vi "Flash Start Live Mode.vi"(8 "error in (no error)":errorcluster, 10 "Camera Settings":T1={"Exposure Time (ms)"=100.0, "Binning"=enum."2x2", "Scan Mode (Flash)"=enum."Fast", "Trigger Mode (Flash)"=enum."Fast", "Frames to Acquire"=1000.0, "Pixel Correction (Flash)"=FALSE} {"Exposure Time (ms)" min=1.0 max=10000.0 step=1.0}, 11 "Orca-Flash 4.0 V2 in":refnum<class "Orca-Flash 4.0 V2.lvclass">) -> (0 "error out":errorcluster, 3 "Orca-Flash 4.0 V2 out":refnum<class "Orca-Flash 4.0 V2.lvclass">)   [LabVIEW 2018, in "Orca-Flash 4.0 V2.lvlib" / "Orca-Flash 4.0 V2.lvclass"]
uses:
  Orca-Flash 4.0 V2.lvclass
  C:/LVCUR/flash-gordon/Hardware/Camera/Camera.lvclass
  Resources/Type Defs/Camera Settings.ctl
  Orca-Flash 4.0 V2.lvclass/Orca-Flash 4.0 V2.ctl
  Resources/GLOBAL/GLOBAL Time-critical.vi
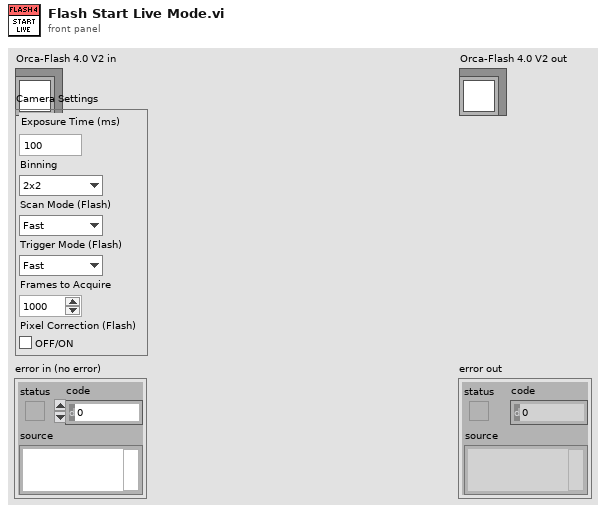
[diagram p1: front panel]
types:
  T1 = typedef "Camera Settings.ctl" = cluster{"Exposure Time (ms)":dbl, "Binning":enum16{"1x1", "2x2", "4x4"}, "Scan Mode (Flash)":enum16{"Fast", "Slow"}, "Trigger Mode (Flash)":enum16{"Fast", "Standard"}, "Frames to Acquire":dbl, "Pixel Correction (Flash)":bool}
  T2 = cluster{"height":i32, "width":i32, "datatype":i32}
  T3 = typedef "Semaphore RefNum" = refnum<k1>
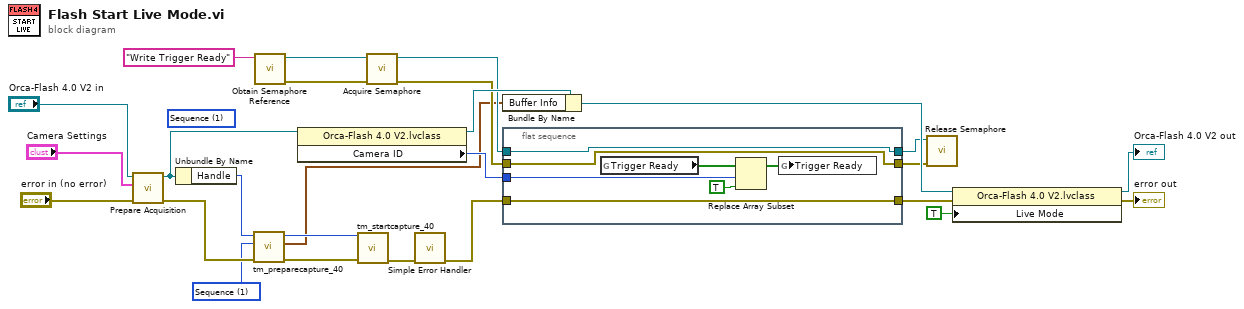
[diagram p0: block diagram]
diagram:
  w4 = 1 items=["Snap", "Sequence"] ("Capture mode")
  (unwired) 1 items=["Snap", "Sequence"] ("Capture mode")
  n1 = call "Prepare Acquisition.vi"("error in (no error)"="error in (no error)", "Flash Settings"="Camera Settings", "Orca-Flash 4.0 in"="Orca-Flash 4.0 V2 in") -> ("error out"=w6:errorcluster, "Orca-Flash 4.0 out"=w16:refnum<class "Orca-Flash 4.0 V2.lvclass">)  [unwired: 7 in]
  n2 = Unbundle By Name(w16) -> ("Handle"=w5:u32)
  n3 = call <userlib>:"tm_preparecapture_40.vi"("error in (no error)"=w6, "Capture mode"=w4, "Handle in"=w5) -> ("error out"=w8:errorcluster, "Buffer Info"=w3:T2, "Handle out"=w7:u32)  [unwired: 5 in, 1 out]
  n4 = call <vilib>:"Obtain Semaphore Reference.vi"("name (unnamed)"="Write Trigger Ready") -> ("error out"=w13:errorcluster, "semaphore"=w14:T3)  [unwired: 4 in, 1 out]
  n5 = property class="Orca-Flash 4.0 V2.lvclass"(reference=w16) -> (reference out=w17:refnum<class "Orca-Flash 4.0 V2.lvclass">, "Camera ID"=w19:i32)  [unwired: 1 in, 1 out]
  n6 = call <userlib>:"tm_startcapture_40.vi"("error in (no error)"=w8, "Handle in"=w7) -> ("error out"=w2:errorcluster)  [unwired: 8 in, 1 out]
  n7 = call <vilib>:"Acquire Semaphore.vi"("error in (no error)"=w13, "semaphore"=w14) -> ("error out"=w9:errorcluster, "semaphore out"=w10:T3)  [unwired: 3 in, 1 out]
  n8 = call <vilib>:"Simple Error Handler.vi"("error in (no error)"=w2) -> ("error out"=w1:errorcluster)  [unwired: 4 in, 4 out]
  n9 = Bundle By Name(cluster=w17, "Buffer Info"=w3) -> (w23:refnum<class "Orca-Flash 4.0 V2.lvclass">)
  n10 = flat-sequence {
    tunnel: w1 -> [w33]
    tunnel: [w33] -> w20
    tunnel: w19 -> [w30]
    tunnel: [w28] -> w12
    tunnel: [w27] -> w11
    tunnel: w10 -> [w28]
    tunnel: w9 -> [w27]
    frame #0 {
      n11 = global read "GLOBAL Time-critical.vi" "Trigger Ready"() -> (w32:bool[])
      n12 = Replace Array Subset(array=w32, new element=TRUE ("new element/subarray"), index=w30) -> (w31:bool[])
      n13 = global write "GLOBAL Time-critical.vi" "Trigger Ready"(w31) -> ()
    }
  }
  n14 = call <vilib>:"Release Semaphore.vi"("error in (no error)"=w11, "semaphore"=w12) -> ()  [unwired: 4 in, 2 out]
  n15 = property class="Orca-Flash 4.0 V2.lvclass"(reference=w23, error in=w20, "Live Mode"=TRUE) -> (reference out=→"Orca-Flash 4.0 V2 out":refnum<class "Orca-Flash 4.0 V2.lvclass">, error out=→"error out":errorcluster)
